vi "Configure Text.vi"(0 "Display State In":T1 caption="State") -> (1 "Show Boolean Text":bool, 2 "Text Array":string[](array[string]))   [LabVIEW 2012, in "Hover Button.xctl"]
doc: "This vi converts the Boolean Text information from the State data to a format needed to write to the Boolean button properties."
uses:
  Hover Button.xctl
  State.ctl
  Button Colors.ctl
  Font Properties.ctl
panel:
  # "This vi reads in the text related State data\nand converts it to the format required for\nthe Boolean button properties"
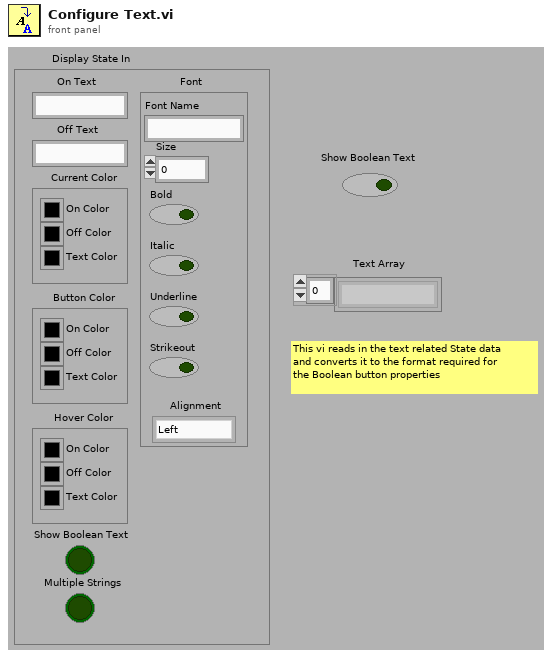
[diagram p1: front panel]
types:
  T1 = typedef "Hover Button.xctl/State.ctl" = cluster{"On Text":string, "Off Text":string, "Current Color":T2, "Button Color":T2, "Hover Color":T2, "Show Boolean Text":bool, "Multiple Strings":bool, "Font":T3}
  T2 = typedef "Hover Button.xctl/Button Colors.ctl" = cluster{"On Color":u32, "Text Color":u32, "Off Color":u32}
  T3 = typedef "Hover Button.xctl/Font Properties.ctl" = cluster{"Font Name":string, "Size":u32, "Bold":bool, "Italic":bool, "Underline":bool, "Strikeout":bool, "Alignment":enum16{"Left", "Center", "Right"}}
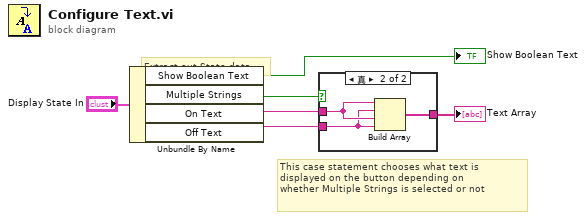
[diagram p0: block diagram]
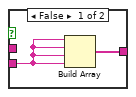
[diagram p2: hidden frame]
diagram:
  # "Extract out State data"
  # "This case statement chooses what text is\ndisplayed on the button depending on\nwhether Multiple Strings is selected or not"
  n1 = Unbundle By Name("Display State In") -> ("Show Boolean Text"=→"Show Boolean Text":bool, "Multiple Strings"=w4:bool, "On Text"=w3:string, "Off Text"=w2:string)
  n2 = case shown="真" w4 {
    tunnel: w3 -> [_ w11]
    tunnel: w2 -> [w7 w10]
    tunnel: [w8 w9] -> w1
    frame False {
      n3 = Build Array(w7, w7, w7, w7) -> (w8:string[])
    }
    frame True {
      n4 = Build Array(w11, w10, w11, w10) -> (w9:string[])
    }
  }
  "Text Array" <- w1
